vi "15_NOV_UPDATE_.vi"() -> ()   [LabVIEW 2020]
panel:
  out "Waveform Chart 2":dbl(graph)
  in  "Save data":bool
  in  "File_name":path=path "saved_data"
  out "Y -axis":string
  out "X -axis":string
  out "SCPI Command":string
  in  "Time interval between iterations (seconds)":dbl
  out "?":cluster{"X":dbl[], "Y":dbl[]}[](graph)
  out "Waveform Chart":dbl(graph)
  out "Measured Output Value":dbl
  in  "SELECT DEVICE":refnum<visa-resource-name>="USB0::0x0957::0x8E18::MY51140695::INSTR"
  out "Resolution":dbl format="%#_6f"
  out "Instantaneous Input Value":dbl format="%#_6f"
  in  "Final Value":dbl
  in  "Initial Value":dbl
  in  "Steps":dbl
  in  "Measure (OUTPUT)":enum16{"Voltage", "Current"}(ring)
  in  "Source":enum16{"Voltage", "Current"}(ring)
  in  "Channel":u16(ring) items=["1", "2"]
  # "1. Include file extension .txt after filename while saving\n\n2. Give unique filename to avoid overwriting data."
  # "(INPUT)"
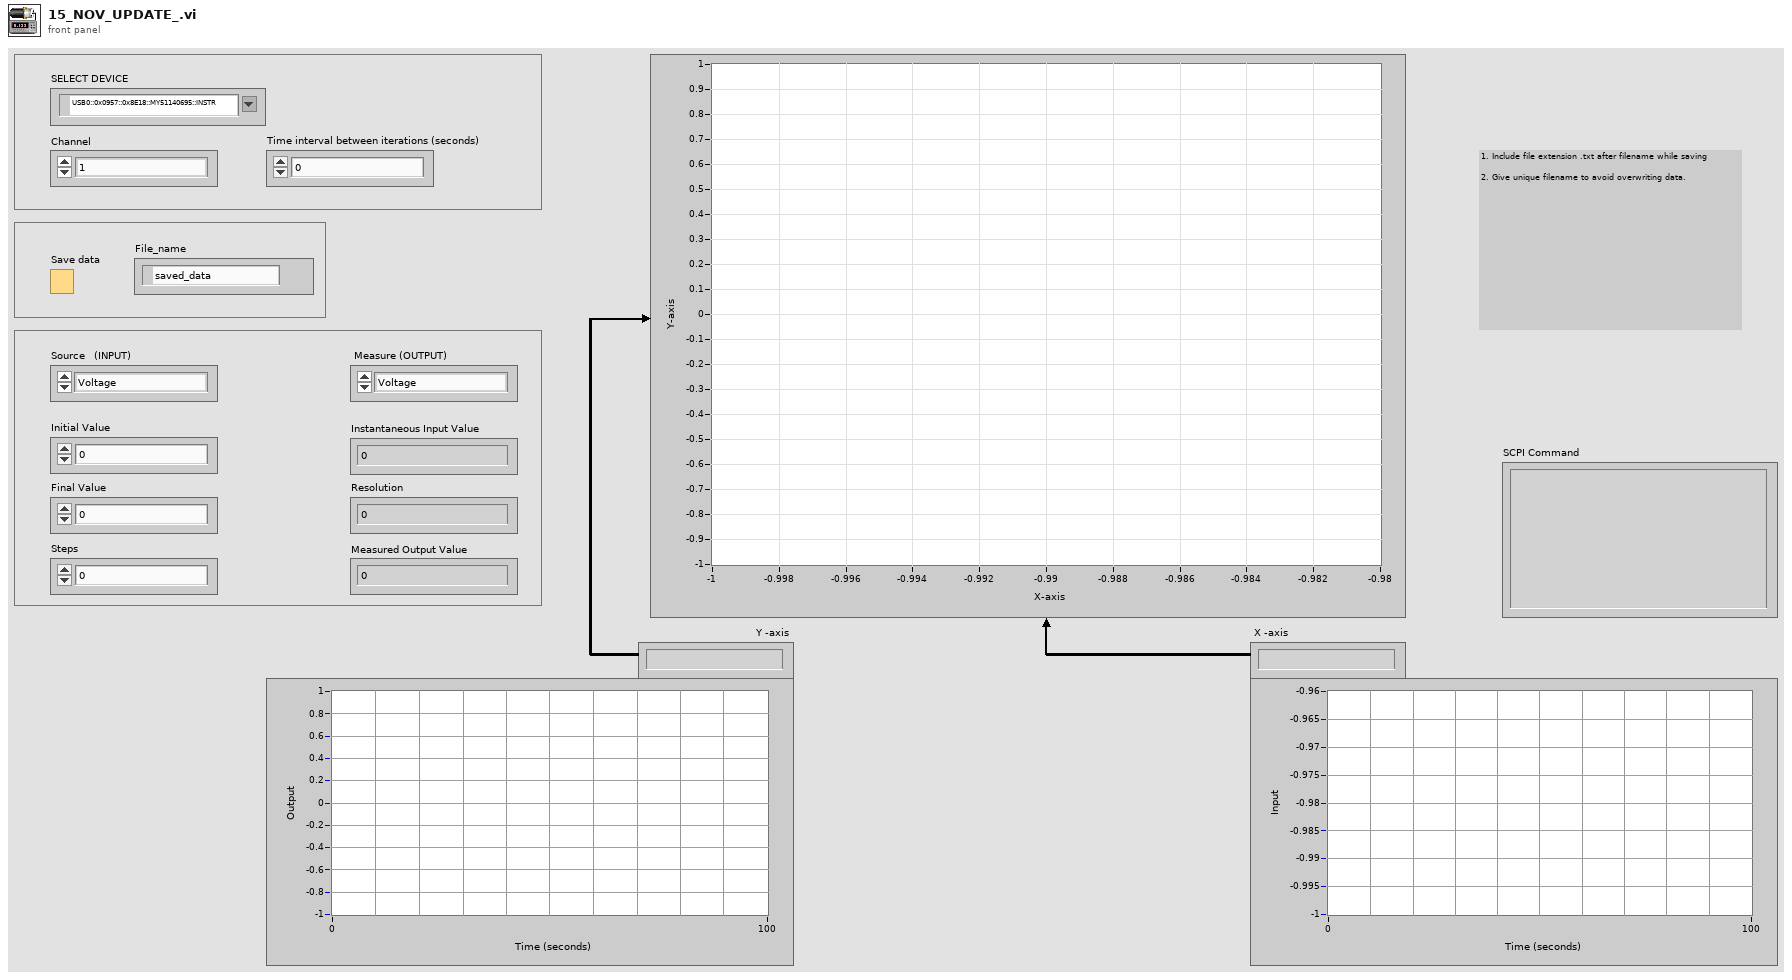
[diagram p1: front panel]
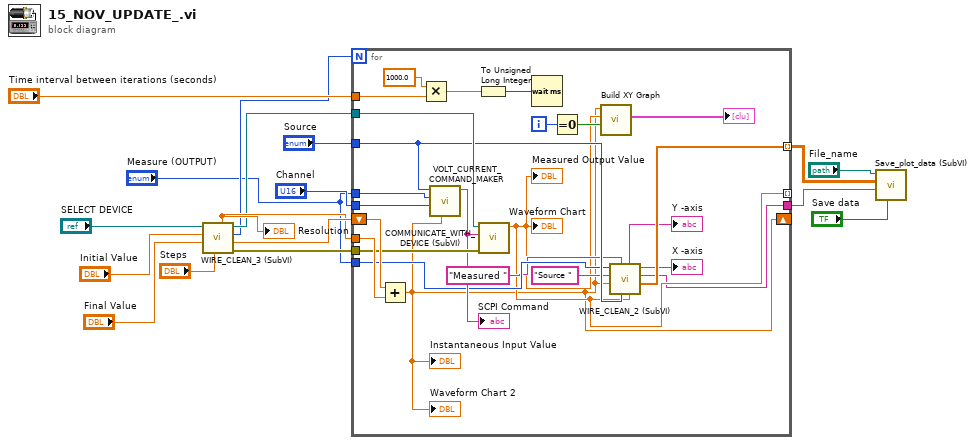
[diagram p0: block diagram]
diagram:
  n1 = call "WIRE_CLEAN_3 (SubVI).vi"("Steps"="Steps", "Final Value"="Final Value", "Initial Value"="Initial Value", "VISA Refnum in"="SELECT DEVICE") -> ("error out"=w8:errorcluster, "Numeric 3"=w14:dbl, "Numeric"=w6:u32, "VISA Refnum out"=w9:refnum<visa-resource-name>, "Numeric 2"=w13:dbl)  [unwired: 3 in]
  "Resolution" <- w13
  n2 = for {
    N: w6 -> [_]
    tunnel: "Channel" -> [w41]
    tunnel: "Source" -> [w28]
    tunnel: "Measure (OUTPUT)" -> [w40]
    tunnel: w13 -> [w38]
    shift-right: [w21] -> _
    shift-left: w14 -> [w39]
    tunnel: w9 -> [w37]
    tunnel: w8 -> [w36]
    tunnel: "Time interval between iterations (seconds)" -> [w33]
    tunnel: "Measure (OUTPUT)" -> [w27]
    tunnel: [w23] -> _ mode=indexing
    tunnel: [w22] -> w3 mode=indexing
    tunnel: [w18] -> w2
    i -> [w35]
    n3 = Add(x=w39, y=w38) -> (x+y=w21:dbl)
    "Instantaneous Input Value" <- w21
    "Waveform Chart 2" <- w21
    n4 = Multiply(x=1000.0, y=w33) -> (x*y=w30:dbl)
    n5 = call "VOLT_CURRENT_COMMAND_MAKER.vi"("Input value"=w21, "Channel"=w41, "Measure (OUTPUT)"=w40, "Source"=w28) -> ("created command"=w29:string)  [unwired: 7 in]
    "SCPI Command" <- w29
    n6 = To Unsigned Long Integer(number=w30) -> (unsigned 32bit integer=w31:u32)
    n7 = call "COMMUNICATE_WITH_DEVICE (SubVI).vi"("error in (no error)"=w36, "created command"=w29, "VISA Refnum in"=w37) -> ("Measured Output Value"=w23:dbl)  [unwired: 7 in, 1 out]
    "Measured Output Value" <- w23
    "Waveform Chart" <- w23
    n8 = Wait (ms)(milliseconds to wait=w31) -> ()  [unwired: 1 out]
    n9 = Equal To 0?(x=w35) -> (x = 0?=w34:bool)
    n10 = call "Build XY Graph"("Reset"=w34, "Y Input"=w23, "X Input"=w21) -> ("XY Graph"=→"?":cluster{"X":dbl[], "Y":dbl[]}[])  [unwired: 7 in, 1 out]
    n11 = call "WIRE_CLEAN_2 (SubVI).vi"("Measured Output Value"=w23, "Source"=w28, "string (\"\")"="Measured " ("string (\"\")"), "Numeric"=w21, "string (\"\") 2"="Source " ("string (\"\")"), "Measure (OUTPUT)"=w27) -> ("Array"=w22:dbl[], "String"=w18:string, "output string 2"=→"X -axis":string, "output string"=→"Y -axis":string)  [unwired: 2 in]
  }
  n12 = call "Save_plot_data (SubVI).vi"("Save data"="Save data", "String"=w2, "Array"=w3, "File_name"="File_name") -> ()  [unwired: 8 in]
